vi "Construct Server Network Messenger.vi"(5 "Log Alias":string, 7 "Log Instance":refnum<class "LoggerReference.lvclass">, 9 "Port":u16, 10 "Connection State Change Callback":refnum<class "IConnectionStateChangeCallback.lvclass">, 11 "Packet Return":refnum<class "IPacket Return.lvclass">) -> (0 "error out":errorcluster, 3 "Network Node":refnum<data-value>)   [LabVIEW 2019, in "Network Messenger.lvlib" / "Network Messenger.lvclass"]
uses:
  <vilib>/gpm_packages/@cs/Network-interface/Source/Network Messenger/Network Messenger.lvclass
  <vilib>/gpm_packages/@cs/Network-interface/Source/MessagingInterfaces/IConnectionStateChangeCallback/IConnectionStateChangeCallback.lvclass
  <vilib>/gpm_packages/@cs/Network-interface/Source/Network Messenger/IPacket Return/IPacket Return.lvclass
  <vilib>/gpm_packages/@cs/event-logger/Source/Composed Log/LoggerReference/LoggerReference.lvclass
  <vilib>/gpm_packages/@cs/Network-interface/Source/Network Messenger/Header Data Packet Return/Header Data Packet Return.lvclass/Header Data Packet Return.ctl
  <vilib>/gpm_packages/@cs/Network-interface/Source/Network Messenger/Write Strategy/Write Strategy.lvclass
  C:/Program Files/National Instruments/LabVIEW 2019/vi.lib/gpm_packages/@cs/Network-interface/Source/MessagingInterfaces/IWriteStrategy/IWriteStrategy.lvclass
  <vilib>/gpm_packages/@cs/Network-interface/Source/Network Messenger/ReadStrategy/ReadStrategy.lvclass
  C:/Program Files/National Instruments/LabVIEW 2019/vi.lib/gpm_packages/@cs/Network-interface/Source/MessagingInterfaces/IReadStrategy/IReadStrategy.lvclass
  <vilib>/gpm_packages/@cs/Network-interface/Source/Network Messenger/Network Messenger.lvclass/Network Messenger.ctl
  <vilib>/gpm_packages/@cs/Network-interface/Source/Create Ref Message/Create Ref Message.lvclass/Create Ref Message.ctl
  <vilib>/ActorFramework/Message Enqueuer/Message Enqueuer.lvclass/Message Enqueuer.ctl
  <vilib>/ActorFramework/Message Enqueuer/Enqueue.vi
  <vilib>/gpm_packages/@cs/Network-interface/Source/Network Messenger/Header Data Packet Return/Header Data Packet Return.lvclass
  C:/Program Files/National Instruments/LabVIEW 2019/vi.lib/gpm_packages/@cs/Network-interface/Source/MessagingInterfaces/IMessageReturnPolicy/IMessageReturnPolicy.lvclass
  <vilib>/gpm_packages/@cs/Network-interface/Source/TCP Interface/TCP Server/TCP Server.lvclass
  C:/Program Files/National Instruments/LabVIEW 2019/vi.lib/gpm_packages/@cs/Network-interface/Source/IConnectionFactory/IConnectionFactory.lvclass
  <vilib>/gpm_packages/@cs/Network-interface/Source/PersistantConnectionHandler/PersistantConnectionHandler/PersistantConnectionHandler.lvclass
  C:/Program Files/National Instruments/LabVIEW 2019/vi.lib/ActorFramework/Actor/Actor.lvclass
  <vilib>/gpm_packages/@cs/Network-interface/Source/Create Ref Message/Create Ref Message.lvclass
  C:/Program Files/National Instruments/LabVIEW 2019/vi.lib/ActorFramework/Message/Message.lvclass
  <vilib>/ActorFramework/Message Priority Queue/Priority Enqueue.vi
  <vilib>/ActorFramework/Actor/Actor.lvclass
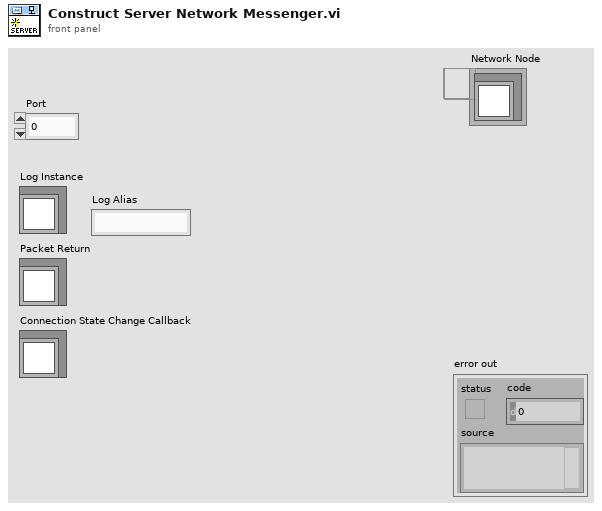
[diagram p1: front panel]
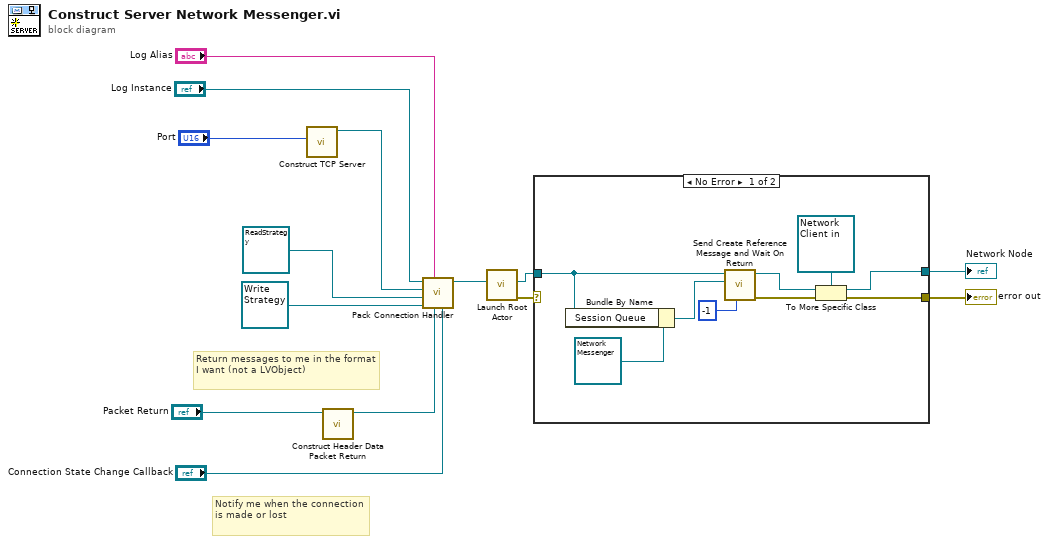
[diagram p0: block diagram]
diagram:
  # "Return messages to me in the format I want (not a LVObject)"
  # "Notify me when the connection is made or lost"
  n1 = call <vilib>:"Construct TCP Server.vi"("Port"="Port") -> ("TCP Server out"=w2:refnum<class "TCP Server.lvclass">)  [unwired: 10 in]
  n2 = call <vilib>:"Construct Header Data Packet Return.vi"("Packet Return"="Packet Return") -> ("Header Data Packet Return out"=w13:refnum<class "Header Data Packet Return.lvclass">)  [unwired: 10 in]
  n3 = call <vilib>:"Pack Connection Handler.vi"("State Change Callback"="Connection State Change Callback", "Message Return Policy"=w13, "Log Alias"="Log Alias", "Write Strategy"=refnum<class "Write Strategy.lvclass"> refnum ("Network Messenger.lvlib:Write Strategy.lvclass"), "Read Strategy"=refnum<class "ReadStrategy.lvclass"> refnum ("Network Messenger.lvlib:ReadStrategy.lvclass"), "Connection Factory Type"=w2, "Log Instance"="Log Instance") -> ("PersistantConnectionHandler out"=w11:refnum<class "PersistantConnectionHandler.lvclass">)  [unwired: 4 in]
  n4 = call <vilib>:"Launch Root Actor.vi"("Actor"=w11) -> ("error out"=w10:errorcluster, "Actor's Enqueuer"=w9:refnum<class "Message Enqueuer.lvclass">)  [unwired: 9 in]
  n5 = case shown="No Error" w10 {
    selector: w10 -> [_ w24]
    tunnel: w9 -> [w22 _]
    tunnel: [w18 _] -> w8
    tunnel: [w17 w24] -> w7
    frame No Error {
      n6 = Bundle By Name(cluster=refnum<class "Network Messenger.lvclass"> refnum ("Network Client in"), "Session Queue"=w22) -> (w23:refnum<class "Network Messenger.lvclass">)
      n7 = call <vilib>:"Send Create Reference Message and Wait On Return.vi"("timeout in ms (-1)"=-1, "Object"=w23, "Message Enqueuer in"=w22) -> ("error out"=w21:errorcluster, "Object Reference"=w20:refnum<data-value>)  [unwired: 7 in]
      n8 = To More Specific Class(target class=refnum<data-value> refnum ("Network Node"), reference=w20, error in=w21) -> (specific class reference=w18:refnum<data-value>, error out=w17:errorcluster)
    }
    frame Error {
    }
  }
  "error out" <- w7
  "Network Node" <- w8
